vi "Read Fisrt Time Series.vi"(8 "error in (no error)":errorcluster, 11 "Readout Charact in":refnum<class "Readout Charact.lvclass">) -> (0 "error out":errorcluster, 2 "Fisrt Time Series":dbl, 3 "Readout Charact out":refnum<class "Readout Charact.lvclass">)   [LabVIEW 2018, in "Readout Charact.lvclass"]
uses:
  Readout Charact.lvclass
  Readout Charact.lvclass/Readout Charact.ctl
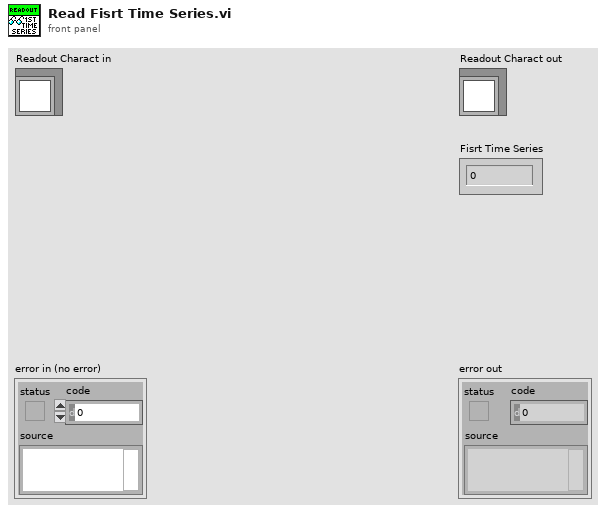
[diagram p1: front panel]
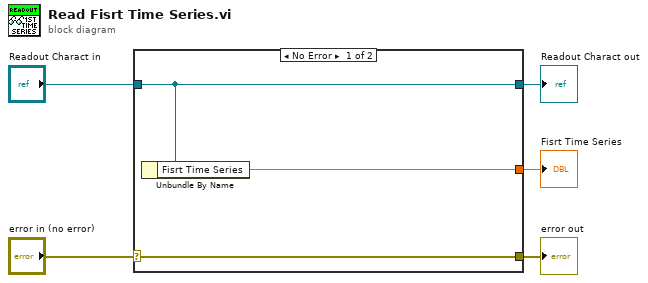
[diagram p0: block diagram]
diagram:
  n1 = case shown="No Error" "error in (no error)" {
    selector: "error in (no error)" -> [w8 w9]
    tunnel: [w8 w9] -> w4
    tunnel: [w7 w10] -> w2
    tunnel: "Readout Charact in" -> [w7 w10]
    tunnel: [w6 _] -> w1
    frame No Error {
      n2 = Unbundle By Name(w7) -> ("Fisrt Time Series"=w6:dbl)
    }
    frame Error {
    }
  }
  "error out" <- w4
  "Readout Charact out" <- w2
  "Fisrt Time Series" <- w1
